vi "DriveModuleOpen.vi"(6 "Magnet Offset (Degrees)":dbl, 7 "ModualNamePrefix":string, 8 "error in":errorcluster, 9 "EncoderCanID":u8, 10 "SpinCanID":u8, 11 "TravelCanID":u8) -> (0 "error out":errorcluster)   [LabVIEW 2025]
uses:
  <vilib>/Rock Robotics/WPI/ThirdParty/REV Robotics/REVLib/Typedef/Spark MAX Idle Mode.ctl
  <vilib>/Rock Robotics/WPI/ThirdParty/REV Robotics/REVLib/SubVI/Public/SPARK Open Brushless.vi
  <vilib>/Rock Robotics/WPI/ThirdParty/REV Robotics/REVLib/SubVI/Public/SPARK Configure Basic Idle Mode.vi
  <vilib>/Rock Robotics/WPI/ThirdParty/REV Robotics/REVLib/SubVI/Public/SPARK Configure Encoder Conversion Factors.vi
  <vilib>/Rock Robotics/WPI/ThirdParty/REV Robotics/REVLib/SubVI/Public/SPARK Configure Basic Ramp Rate.vi
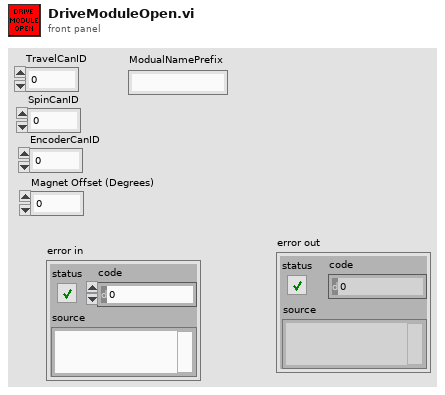
[diagram p1: front panel]
types:
  T1 = typedef "Spark MAX Idle Mode.ctl" = enum16{"Coast", "Brake"}
  T2 = typedef "WPI_MotorControlDeviceRef.ctl" = cluster{"DeviceStatus":errorcluster, "Type":T3, "PWM":cluster{"PWM Channel":T4, "DeadBand":T5}, "CAN":cluster{"Device Number":u8, "SetOutput VI Ref":variant, "GetOutput VI Ref":variant, "Enable VI Ref":variant, "Disable VI Ref":variant, "Data":variant}, "Invert":bool, "DIO PWM":cluster{"PWM \"Enable\" Channel":T4, "DIOChannel":T6, "PWM Rate":dbl}}
  T3 = typedef "WPI_MotorControlType.ctl" = enum16{"PWM", "CAN", "DIO PWM"}
  T4 = typedef "FPGA_DIOPWMChannel.ctl" = enum8{"PWM 0", "PWM 1", "PWM 2", "PWM 3", "PWM 4", "PWM 5", "PWM 6", "PWM 7", "PWM 8", "PWM 9", "PWM MXP 0", "PWM MXP 1", "PWM MXP 2", "PWM MXP 3", "PWM MXP 4", "PWM MXP 5", "PWM MXP 6", "PWM MXP 7", "PWM MXP 8", "PWM MXP 9", "Invalid"}
  T5 = typedef "WPI_PWMDeadband.ctl" = cluster{"Name":string, "maxPositivePwm":i32, "minPositivePwm":i32, "centerPwm":i32, "maxNegativePwm":i32, "minNegativePwm":i32, "angularRange":u16}
  T6 = typedef "FPGA_DIOChannel.ctl" = enum8{"DIO 0", "DIO 1", "DIO 2", "DIO 3", "DIO 4", "DIO 5", "DIO 6", "DIO 7", "DIO 8", "DIO 9", "DIO MXP 0", "DIO MXP 1", "DIO MXP 2", "DIO MXP 3", "DIO MXP 4", "DIO MXP 5", "DIO MXP 6", "DIO MXP 7", "DIO MXP 8", "DIO MXP 9", "DIO MXP 10", "DIO MXP 11", "DIO MXP 12", "DIO MXP 13", "DIO MXP 14", "DIO MXP 15", "SPI Port CS1", "SPI Port CS2", "SPI Port CS3", "SPI Port MISO", "SPI Port MOSI", "Invalid"}
  T7 = typedef "DeviceReference.ctl" = cluster{"CANbus Name":string, "Device Encoding":u32, "Device Name":string}
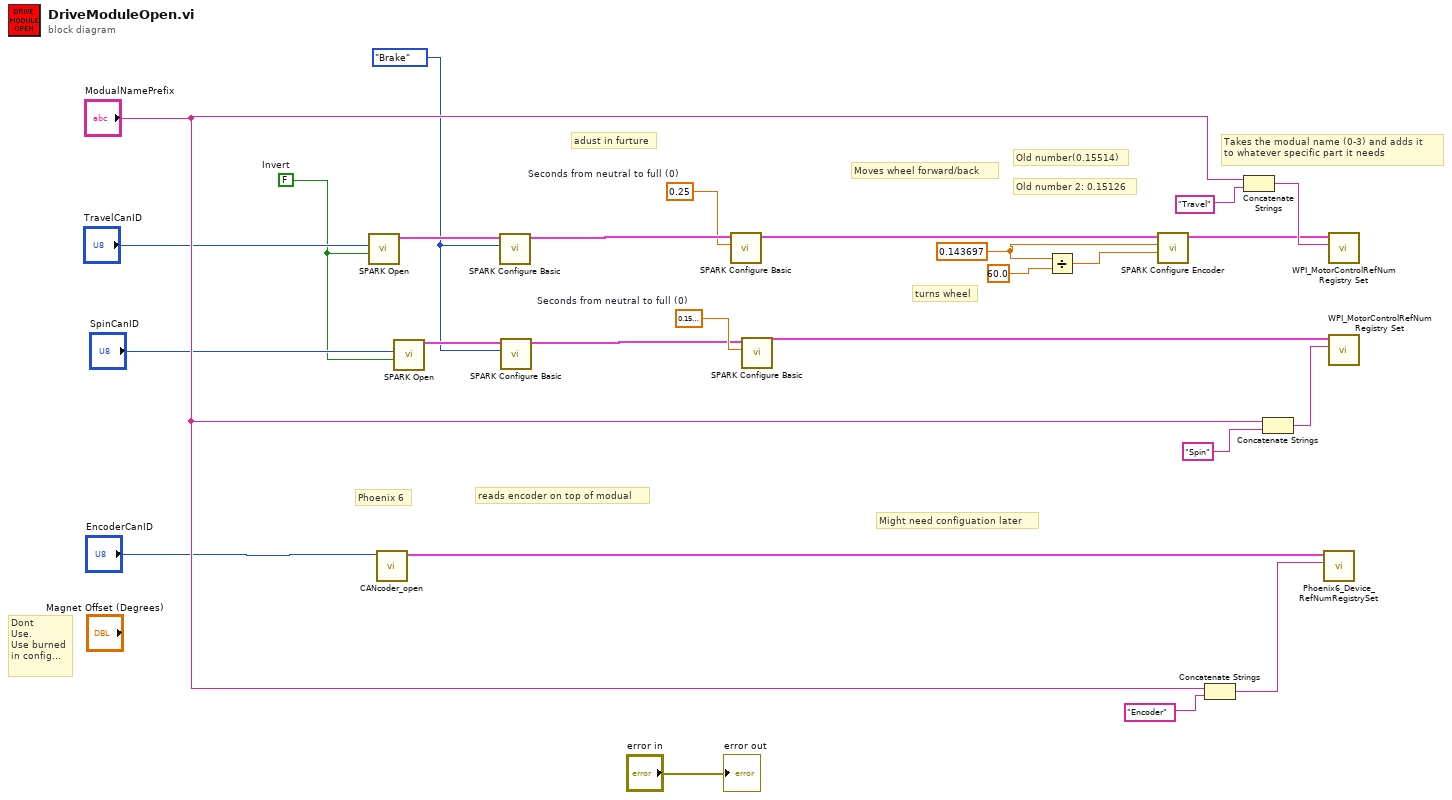
[diagram p0: block diagram]
diagram:
  w6 = sgl 0.15  # Seconds from neutral to full (0)
  w15 = sgl 0.25  # Seconds from neutral to full (0)
  w7 = Spark_MAX_Idle_Mode."Brake" ("Idle Mode")
  w13 = 0.143697 ("Position Factor (1)")
  w9 = FALSE  # Invert
  # "Phoenix 6"
  # "Dont\nUse.\nUse burned\nin config..."
  # "adust in furture"
  # "Old number 2: 0.15126"
  # "Old number(0.15514)"
  # "reads encoder on top of modual"
  # "turns wheel"
  # "Moves wheel forward/back"
  # "Might need configuation later"
  # "Takes the modual name (0-3) and adds it \nto whatever specific part it needs"
  n1 = call-poly <vilib>:"SPARK Open.vi"("Invert"=w9, "Device Number"="TravelCanID") -> ("MotorControlDeviceRef"=w17:T2)  [unwired: 8 in, 1 out]
  n2 = call <vilib>:"CANcoder_open.vi"("Device ID"="EncoderCanID") -> ("DeviceReference 2"=w2:T7)  [unwired: 9 in, 1 out]
  n3 = call-poly <vilib>:"SPARK Open.vi"("Invert"=w9, "Device Number"="SpinCanID") -> ("MotorControlDeviceRef"=w8:T2)  [unwired: 8 in, 1 out]
  n4 = call-poly <vilib>:"SPARK Configure Basic.vi"("Idle Mode"=w7, "MotorControlDeviceRef in"=w17) -> ("MotorControlDeviceRef out"=w16:T2)  [unwired: 8 in, 1 out]
  n5 = call-poly <vilib>:"SPARK Configure Basic.vi"("Idle Mode"=w7, "MotorControlDeviceRef in"=w8) -> ("MotorControlDeviceRef out"=w5:T2)  [unwired: 8 in, 1 out]
  n6 = call-poly <vilib>:"SPARK Configure Basic.vi"("Seconds from neutral to full (0)"=w15, "MotorControlDeviceRef in"=w16) -> ("MotorControlDeviceRef"=w14:T2)  [unwired: 8 in, 1 out]
  n7 = call-poly <vilib>:"SPARK Configure Basic.vi"("Seconds from neutral to full (0)"=w6, "MotorControlDeviceRef in"=w5) -> ("MotorControlDeviceRef"=w4:T2)  [unwired: 8 in, 1 out]
  n8 = Divide(x=w13, y=60.0) -> (x/y=w12:dbl)
  n9 = call-poly <vilib>:"SPARK Configure Encoder.vi"("Velocity Conversion Factor"=w12, "Position Conversion Factor"=w13, "MotorControlDeviceRef in"=w14) -> ("MotorControlDeviceRef out"=w11:T2)  [unwired: 7 in, 1 out]
  n10 = Concatenate Strings("ModualNamePrefix", "Encoder" ("refnum name")) -> (w1:string)
  n11 = Concatenate Strings("ModualNamePrefix", "Travel" ("refnum name")) -> (w25:string)
  n12 = Concatenate Strings("ModualNamePrefix", "Spin" ("refnum name")) -> (w23:string)
  n13 = call <vilib>:"Phoenix6_Device_RefNumRegistrySet.vi"("refnum name"=w1, "DeviceReference"=w2) -> ()  [unwired: 8 in, 2 out]
  n14 = call <vilib>:"WPI_MotorControlRefNum Registry Set.vi"("refnum name"=w25, "MotorControlDevRef"=w11) -> ()  [unwired: 8 in, 2 out]
  n15 = call <vilib>:"WPI_MotorControlRefNum Registry Set.vi"("refnum name"=w23, "MotorControlDevRef"=w4) -> ()  [unwired: 8 in, 2 out]
  "error out" <- "error in"
